vi "S706 Parameter senden OSPrompt.vi"(8 "Fehler (Eingang)":errorcluster, 10 "SDO object in":refnum<k20>, 11 "Dateipfad (Dialog verwenden)":path) -> (0 "error out":errorcluster)   [LabVIEW 2014]
uses:
  <vilib>/CANopenLib/CANOPEN.llb/CANopen SDO Write [U8].vi
  <vilib>/CANopenLib/CANOPEN.llb/CANopen SDO Read [I32].vi
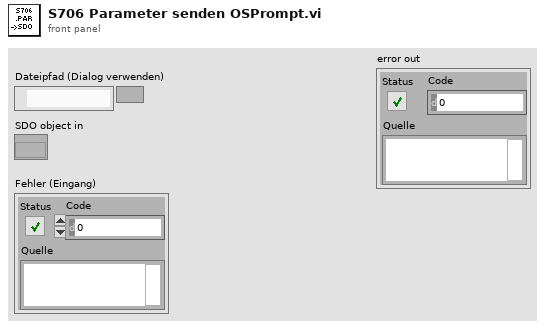
[diagram p1: front panel]
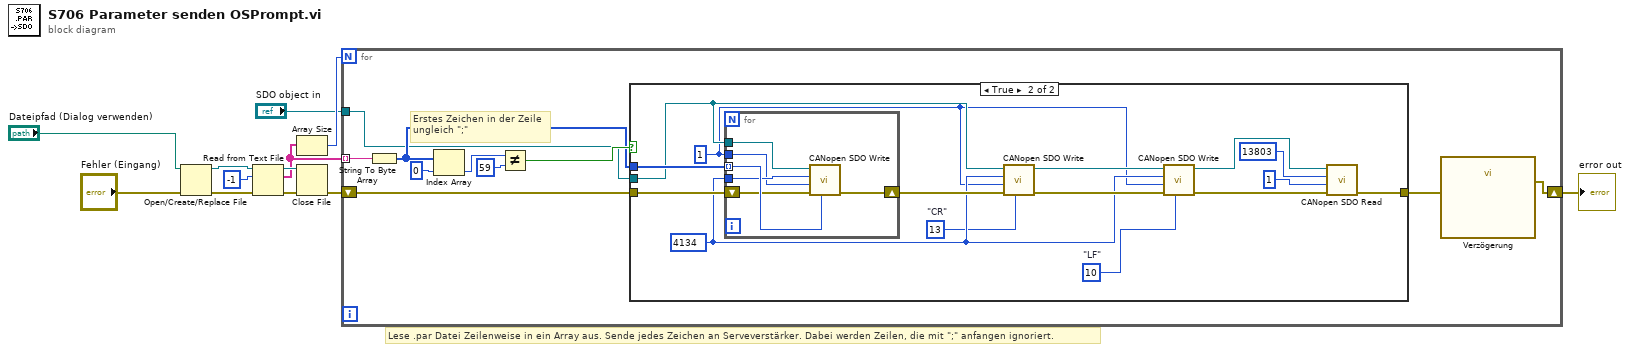
[diagram p0: block diagram]
diagram:
  # "Lese .par Datei Zeilenweise in ein Array aus. Sende jedes Zeichen an Serveverstärker. Dabei werden Zeilen, die mit \";\" anfangen ignoriert."
  n1 = Open/Create/Replace File(file path (use dialog)="Dateipfad (Dialog verwenden)", error in="Fehler (Eingang)") -> (refnum out=w12:refnum<file>, error out=w2:errorcluster)  [unwired: 4 in, 1 out]
  n2 = Read from Text File(file (use dialog)=w12, count=-1 ("Anzahl"), error in=w2) -> (refnum out=w10:refnum<file>, text=w7:string[], error out=w9:errorcluster)  [unwired: 1 in, 1 out]
  n3 = Array Size(array=w7) -> (size(s)=w8:i32)
  n4 = Close File(refnum=w10, error in=w9) -> (error out=w5:errorcluster)  [unwired: 1 out]
  n5 = for {
    N: w8 -> [_]
    tunnel: w7 -> [w22] mode=indexing
    tunnel: "SDO object in" -> [w16]
    shift-right: [w13] -> w4
    shift-left: w5 -> [w15]
    # "Erstes Zeichen in der Zeile\nungleich \";\""
    n6 = String To Byte Array(string=w22) -> (unsigned byte array=w17:u8[])
    n7 = Index Array(array=w17, index=0 ("Index")) -> (element=w18:u8)
    n8 = Not Equal?(x=w18, y=u8 59) -> (x != y?=w20:bool)
    n9 = case shown="True" w20 {
      tunnel: w17 -> [_ w38]
      tunnel: w16 -> [_ w36]
      tunnel: w15 -> [w23 w37]
      tunnel: [w23 w24] -> w14
      frame False {
      }
      frame True {
        w29 = u8 10  # "LF"
        w30 = u8 13  # "CR"
        w31 = u8 1 ("object sub-index (0)")
        w32 = u16 4134 ("object index")
        n10 = for {
          tunnel: w38 -> [w44] mode=indexing
          tunnel: w36 -> [w43]
          shift-right: [w41] -> w33
          shift-left: w37 -> [w42]
          tunnel: w32 -> [w40]
          tunnel: w31 -> [w39]
          n11 = call-poly <vilib>:"CANopen SDO Write.vi"("U8 data"=w44, "error in (no error)"=w42, "object sub-index (0)"=w39, "object index"=w40, "SDO object in"=w43) -> ("error out"=w41:errorcluster)  [unwired: 4 in, 2 out]
        }
        n12 = call-poly <vilib>:"CANopen SDO Write.vi"("U8 data"=w30, "error in (no error)"=w33, "object sub-index (0)"=w31, "object index"=w32, "SDO object in"=w36) -> ("error out"=w34:errorcluster, "SDO object out"=w35:refnum<k20>)  [unwired: 4 in, 1 out]
        n13 = call-poly <vilib>:"CANopen SDO Write.vi"("U8 data"=w29, "error in (no error)"=w34, "object sub-index (0)"=w31, "object index"=w32, "SDO object in"=w35) -> ("error out"=w28:errorcluster, "SDO object out"=w27:refnum<k20>)  [unwired: 4 in, 1 out]
        n14 = call-poly <vilib>:"CANopen SDO Read.vi"("error in (no error)"=w28, "object sub-index (0)"=u8 1, "object index"=u16 13803, "SDO object in"=w27) -> ("error out"=w24:errorcluster)  [unwired: 4 in, 3 out]
      }
    }
    n15 = call "Verzögerung"("error in (no error)"=w14) -> ("error out"=w13:errorcluster)  [unwired: 10 in]
  }
  "error out" <- w4
